vi "Get Table Values.vi"(8 "error in (no error)":errorcluster, 11 "Weather Data":T1[](array[typedef])) -> (0 "error out":errorcluster, 3 "Table Values":string[][](array[string]))   [LabVIEW 2023, in "Weather Monitor Views.lvlib"]
doc: "Converts an array of weather data clusters into an array of strings for displaying in a table."
uses:
  Weather Monitor Views.lvlib
  Application/Weather Data.ctl
  Application/Weather Data.lvlib
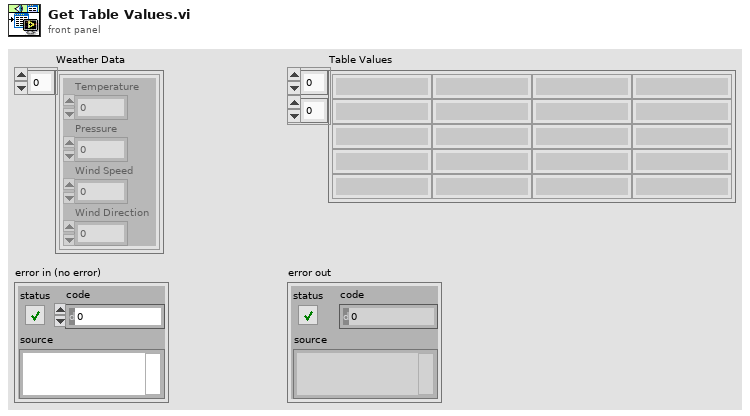
[diagram p1: front panel]
types:
  T1 = typedef "Weather Data.lvlib/Weather Data.ctl" = cluster{"Temperature":dbl, "Pressure":dbl, "Wind Speed":dbl, "Wind Direction":dbl}
  T2 = cluster{"Temperature":string, "Pressure":string, "Wind Speed":string, "Wind Direction":string}
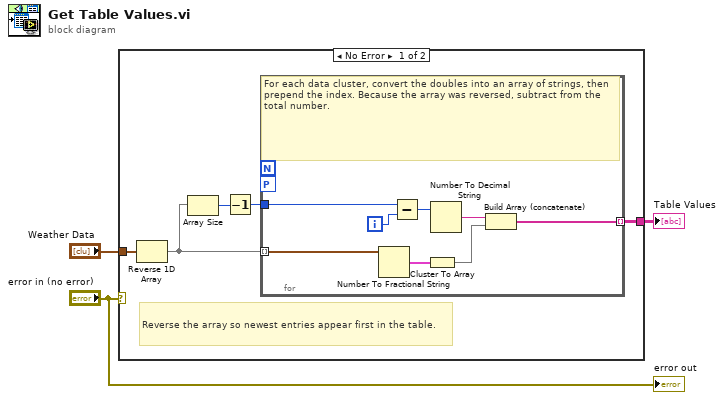
[diagram p0: block diagram]
diagram:
  n1 = case shown="No Error" "error in (no error)" {
    tunnel: "Weather Data" -> [w8 _]
    tunnel: [w7 _] -> w2
    frame No Error {
      # "Reverse the array so newest entries appear first in the table."
      n2 = Reverse 1D Array(array=w8) -> (reversed array=w4:T1[])
      n3 = Array Size(array=w4) -> (size(s)=w6:i32)
      n4 = Decrement(x=w6) -> (x-1=w5:i32)
      n5 = for {
        tunnel: w4 -> [w9] mode=indexing
        tunnel: [w13] -> w7 mode=indexing
        tunnel: w5 -> [w11]
        workers-P: _ -> [_]
        i -> [w16]
        # "For each data cluster, convert the doubles into an array of strings, then prepend the index. Because the array was reversed, subtract from the total number."
        n6 = Number To Fractional String(number=w9) -> (F-format string=w10:T2)  [unwired: 3 in]
        n7 = Subtract(x=w11, y=w16) -> (x-y=w12:i32)
        n8 = Cluster To Array(cluster=w10) -> (array=w14:string[])
        n9 = Number To Decimal String(number=w12) -> (decimal integer string=w15:string)  [unwired: 1 in]
        n10 = Build Array (concatenate)(w15, w14) -> (w13:string[])
      }
    }
    frame Error {
    }
  }
  "Table Values" <- w2
  "error out" <- "error in (no error)"
